vi "Theta Hypotenuse.vi"(2 "x value":dbl=0.1, 3 "y value":dbl=0.1) -> (0 "Theta":dbl, 1 "Hypotenuse":dbl)   [LabVIEW 2019]
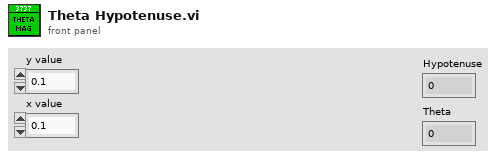
[diagram p1: front panel]
types:
  T1 = cluster{"[0]":dbl, "[1]":dbl, "[2]":dbl, "[3]":dbl, "[4]":dbl, "[5]":dbl, "[6]":dbl, "[7]":dbl, "[8]":dbl}
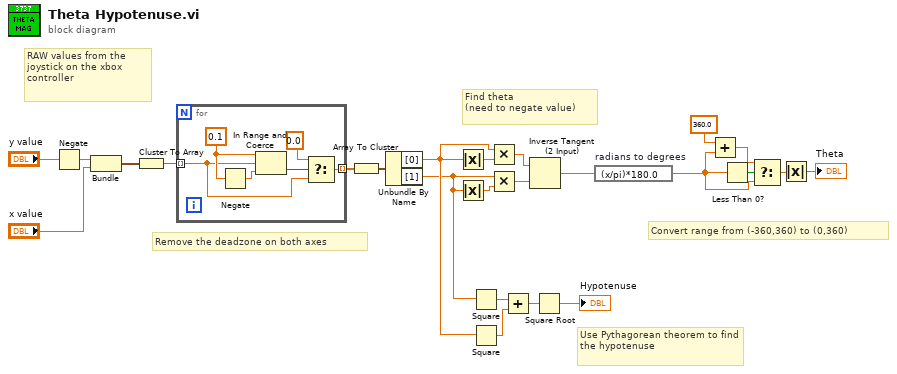
[diagram p0: block diagram]
diagram:
  # "Use Pythagorean theorem to find the hypotenuse"
  # "Convert range from (-360,360) to (0,360)"
  # "Find theta\n(need to negate value)"
  # "Remove the deadzone on both axes"
  # "RAW values from the joystick on the xbox controller"
  n1 = Negate(x="y value") -> (-x=w1:dbl)
  n2 = Bundle(w1, "x value"="x value") -> (w21:cluster{dbl, "x value":dbl})  [unwired: 1 in]
  n3 = Cluster To Array(cluster=w21) -> (array=w22:dbl[])
  n4 = for {
    tunnel: w22 -> [w26] mode=indexing
    tunnel: [w25] -> w20 mode=indexing
    w28 = 0.1 ("lower limit")
    n5 = Negate(x=w28) -> (-x=w29:dbl)
    n6 = In Range and Coerce(upper limit=w28, x=w26, lower limit=w29) -> (In Range?=w30:bool)  [unwired: 1 out]
    n7 = Select(t=0.0, s=w30, f=w26) -> (s? t:f=w25:dbl)
  }
  n8 = Array To Cluster(array=w20) -> (cluster=w19:T1)
  n9 = Unbundle By Name(w19) -> ("[0]"=w4:dbl, "[1]"=w3:dbl)
  n10 = Absolute Value(x=w4) -> (abs(x)=w17:dbl)
  n11 = Absolute Value(x=w3) -> (abs(x)=w18:dbl)
  n12 = Square(x=w3) -> (x^2=w8:dbl)
  n13 = Square(x=w4) -> (x^2=w7:dbl)
  n14 = Multiply(x=w4, y=w17) -> (x*y=w15:dbl)
  n15 = Multiply(x=w3, y=w18) -> (x*y=w16:dbl)
  n16 = Add(x=w8, y=w7) -> (x+y=w6:dbl)
  n17 = Inverse Tangent (2 Input)(1:w16, 2:w15) -> (0:w2:dbl)
  n18 = Square Root(x=w6) -> (sqrt(x)=→"Hypotenuse":dbl)
  n19 = expression code="(x/pi)*180.0" "radians to degrees"(w2) -> (w11:dbl)
  n20 = Add(x=360.0, y=w11) -> (x+y=w13:dbl)
  n21 = Less Than 0?(x=w11) -> (x < 0?=w14:bool)
  n22 = Select(t=w13, s=w14, f=w11) -> (s? t:f=w10:dbl)
  n23 = Absolute Value(x=w10) -> (abs(x)=→"Theta":dbl)
